vi "AppleScript Global Data.vi"() -> ()   [LabVIEW 2017, in "Apple script.lvlib"]
uses:
  Apple script.lvlib
panel:
  out "Array":void[](array[numeric])
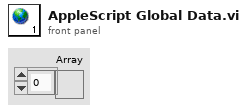
[diagram p1: front panel]
diagram:
